vi "解析寄电器.vi"(8 "error in (no error)":errorcluster caption="错误输入（无错误）", 11 "寄存器in":u16[](array[numeric])) -> (0 "error out":errorcluster caption="错误输出", 1 "分解后报文out":string[](array[string]), 2 "原始报文out":string, 3 "启动信号out":i32)   [LabVIEW 2020]
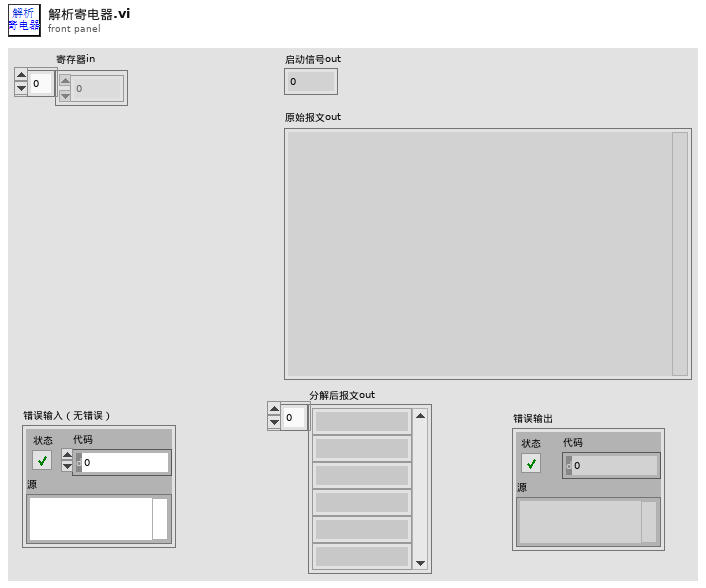
[diagram p1: front panel]
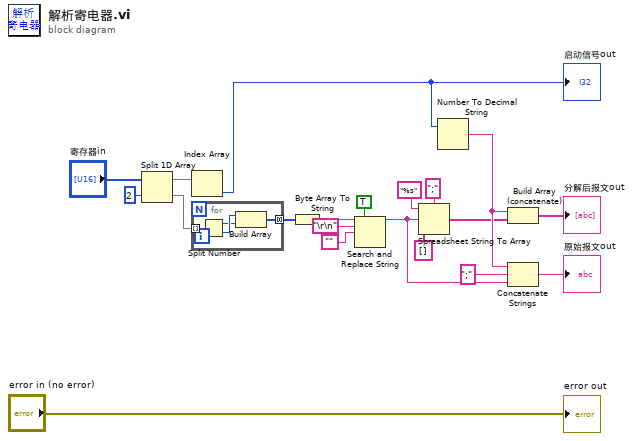
[diagram p0: block diagram]
diagram:
  n1 = Split 1D Array(array="寄存器in", index=2 ("索引")) -> (first subarray=w19:u16[], second subarray=w17:u16[])
  n2 = Index Array(array=w19) -> (element=w7:u16)  [unwired: 1 in]
  "启动信号out" <- w7
  n3 = for {
    tunnel: w17 -> [w24] mode=indexing
    tunnel: [w21] -> w16 mode=concatenating
    n4 = Split Number(x=w24) -> (hi(x)=w22:u8, lo(x)=w23:u8)
    n5 = Build Array(w23, w22) -> (w21:u8[])
  }
  n6 = Byte Array To String(unsigned byte array=w16) -> (string=w11:string)
  n7 = Search and Replace String(replace all?=TRUE ("替换全部？(F)"), input string=w11, search string="\r\n", replace string="") -> (result string=w5:string)  [unwired: 4 in, 3 out]
  n8 = Spreadsheet String To Array(delimiter (Tab)=";" ("分隔符(Tab)"), format string="%s" ("格式字符串"), spreadsheet string=w5, array type (2D Dbl)=string[] []) -> (array=w2:string[])
  n9 = Number To Decimal String(number=w7) -> (decimal integer string=w3:string)  [unwired: 1 in]
  n10 = Build Array (concatenate)(w3, w2) -> (→"分解后报文out":string[])
  n11 = Concatenate Strings(w3, ";" ("字符串"), w5) -> (→"原始报文out":string)
  "error out" <- "error in (no error)"
